vi "pulse from memory 16spc_v3.vi"(7 "stop this pulse":bool, 8 "run":bool=TRUE, 9 "referenses":T3={"clock x2"="IO Socket\\Data Clock 2x", "Memory In"="pulse on memory"}, 10 "start this pulse":bool, 11 "PDW":T1={"PW"=0, "frequency shift"=0.0, "amp"=0.9999923706054688, "mode type"=enum."CW", "mode depth"=0, "mode filter"=0, "phase shift"=0.0, "pulse shape filter"=0} {"frequency shift" format="%#_12f"}) -> (1 "free DDS":bool, 2 "output valid":bool=TRUE, 3 "IQ_out":T4[](array[typedef]))   [LabVIEW 2021]
uses:
  <instrlib>/_niInstr/DSP/v1/Shared/Public/IQ Data.ctl
  pulse_tx_vis/pdw.ctl
  pulse_tx_vis/CTL/mode_type.ctl
  <instrlib>/_niInstr/DSP/v1/FPGA/Public/Sub VIs/Data Conversion/U32 to IQ - 1 spc - S18.1.vi
  <instrlib>/FlexRIO/API/UsrFpgaDsp/v1/FPGA/HbInt/UsrFpgaDspHbIntIQ_8Cps_1xOC_BWper2_96dB.vi
  <instrlib>/FlexRIO/API/UsrFpgaDsp/v1/FPGA/HbInt/UsrFpgaDspHbIntIQ_4Cps_1xOC_BWper2_89dB.vi
  <instrlib>/FlexRIO/API/UsrFpgaDsp/v1/FPGA/HbInt/UsrFpgaDspHbIntIQ_2Cps_1xOC_BWper2_89dB.vi
  <vilib>/rvi/DataTransferAndStorage/Container/Common/niFpgaContainerExecOnDevCompGetState.vi
  <vilib>/rvi/Emulation/niFpgaEmulationIsFPGAContextNoSignature.vi
  <vilib>/rvi/DataTransferAndStorage/Container/Common/niFpgaContainerGetUniqueNameForEmu.vi
  <vilib>/rvi/Emulation/niFpgaProcessEmulError.vi
  <vilib>/rvi/Emulation/niFpgaSctlEmulationGetInTimedLoop.vi
  <vilib>/rvi/errors/nirviReportUnexpectedCaseInternalError (U32).vi
  <vilib>/rvi/Memory/Memory_Emulation/niFpgaMemoryEmulationCacheClearOnFirstRun.vi
  <vilib>/rvi/Memory/Memory_Emulation/nirvimemoryEmulationManagerCache_MakeExclusive.vi
  <vilib>/rvi/Memory/Memory_Emulation/niFpgaMemoryEmulationValidateCache.vi
  <vilib>/rvi/Memory/Memory_Emulation/nirvimemoryEmulationManagerCache_InsertValue.vi
  <vilib>/Utility/error.llb/Clear Errors.vi
  <vilib>/rvi/Memory/Memory_Emulation/nirvimemoryEmulationManagerCache_ReleaseExclusive.vi
  <vilib>/rvi/Memory/Memory_Emulation/nirvimemoryEmulationManagerCache_GetValue.vi
  <vilib>/rvi/Memory/Memory_Emulation/nirvimemoryEmulationManagerCache_SetValue.vi
  <vilib>/rvi/Emulation/niFpgaSctlEmulationResourceMgr.vi
  <instrlib>/FlexRIO/API/UsrFpgaDsp/v1/FPGA/HbInt/UsrFpgaDspHbIntIQ_1Spc_2xOC_BWper2_89dB.vi
  <instrlib>/FlexRIO/API/UsrFpgaDsp/v1/FPGA/HbInt/UsrFpgaDspHbIntIQ_2Spc_2xOC_BWper2_89dB.vi
  <instrlib>/FlexRIO/API/UsrFpgaDsp/v1/FPGA/HbInt/UsrFpgaDspHbIntIQ_4Spc_2xOC_BWper2_89dB.vi
  <instrlib>/FlexRIO/API/UsrFpgaDsp/v1/FPGA/HbInt/UsrFpgaDspHbIntIQ_8Spc_2xOC_BWper2_89dB.vi
  <instrlib>/_niInstr/DSP/v1/FPGA/Public/Sub VIs/Frequency Shift/Frequency Shift - 16 spc.vi
  <instrlib>/_niInstr/Basic Elements/v1/FPGA/Private/Count Up U32.vi
  <instrlib>/_niInstr/Basic Elements/v1/FPGA/Private/Count Up U16.vi
  <vilib>/rvi/DataTransferAndStorage/Container/XNode/niFpgaContainer.xnode
  <vilib>/rvi/Memory/Memory_Emulation/niFpgaMemoryEmulationRefIn.vi
  <instrlib>/_niInstr/DSP/v1/Shared/niInstr DSP v1 Shared.lvlib
  <instrlib>/_niInstr/DSP/v1/FPGA/niInstr DSP v1 FPGA.lvlib
  <instrlib>/_niInstr/Basic Elements/v1/FPGA/niInstr Basic Elements v1 FPGA.lvlib
  <instrlib>/FlexRIO/API/UsrFpgaDsp/v1/FPGA/HbInt/UsrFpgaDsp HbInt v1 FPGA.lvlib
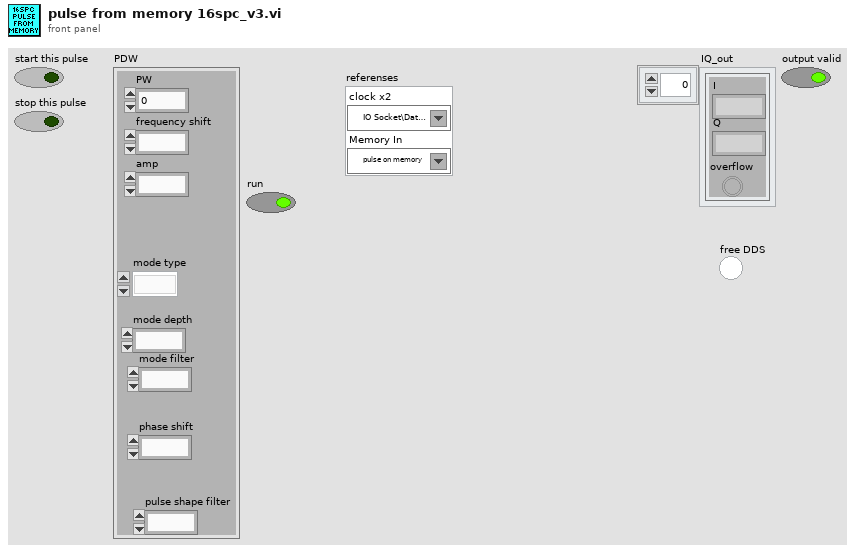
[diagram p1: front panel]
types:
  T1 = typedef "pdw.ctl" = cluster{"PW":u32, "frequency shift":fxp<+/-,48,0>, "amp":fxp<+/-,18,1>, "mode type":T2, "mode depth":u32, "mode filter":u8, "phase shift":fxp<+/-,16,1>, "pulse shape filter":u8}
  T2 = typedef "mode_type.ctl" = enum8{"CW", "from memory 1", "NC - cw", "LFM", "BPSK", "QPSK"}
  T3 = cluster{"clock x2":refnum<k21>, "Memory In":refnum<k21>}
  T4 = typedef "niInstr DSP v1 Shared.lvlib/IQ Data.ctl" = cluster{"I":fxp<+/-,18,1>, "Q":fxp<+/-,18,1>, "overflow":bool}
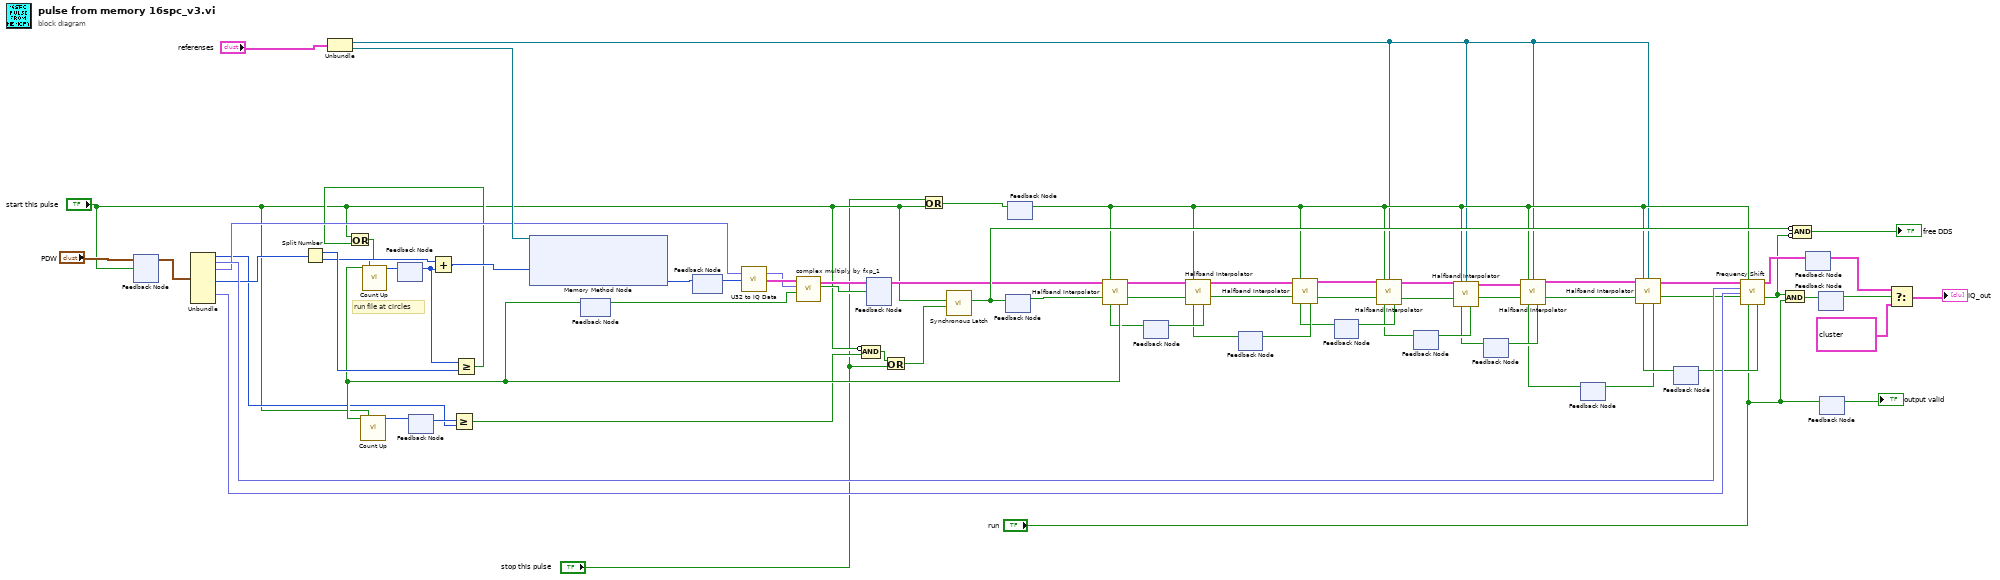
[diagram p0: block diagram]
diagram:
  # "run file at circles"
  n1 = feedback #1() -> (w65:T1)  [unwired: 1 in]
  n2 = feedback-in #1("PDW", "start this pulse") -> ()
  n3 = Unbundle(w65) -> ("PW"=w31:u32, "frequency shift"=w71:fxp<+/-,48,0>, "amp"=w59:fxp<+/-,18,1>, "mode depth"=w37:u32, "phase shift"=w70:fxp<+/-,16,1>)  [unwired: 3 out]
  n4 = Split Number(x=w37) -> (hi(x)=w64:u16, lo(x)=w58:u16)
  n5 = Unbundle("referenses") -> ("clock x2"=w13:refnum<k21>, "Memory In"=w67:refnum<k21>)
  n6 = feedback #2() -> (w56:u16)  [unwired: 1 in]
  n7 = feedback #3() -> (w32:u32)  [unwired: 1 in]
  n8 = Add(x=w58, y=w56) -> (x+y=w55:u16)
  n9 = Greater Or Equal?(x=w32, y=w31) -> (x >= y?=w30:bool)
  n10 = Greater Or Equal?(x=w56, y=w64) -> (x >= y?=w34:bool)
  n11 = Or(x="start this pulse", y=w34) -> (x .or. y?=w35:bool)
  n12 = xnode ("Memory Method Node")("Address"=w55, "Memory In"=w67) -> ("Data"=w74:u32)  [unwired: 1 out]
  n13 = feedback #4() -> (w60:bool)  [unwired: 1 in]
  n14 = feedback #5() -> (w73:u32)  [unwired: 1 in]
  n15 = feedback-in #5(w74) -> ()
  n16 = call-poly <instrlib>:"U32 to IQ Data.vi"("U32 data"=w73) -> ("IQ data"=w62:T4)  [unwired: 14 in]
  n17 = call "complex multiply by fxp_1.vi"("input valid"=w60, "amp"=w59, "IQ data"=w62) -> ("data valid"=w63:bool, "output cluster"=w61:T4)  [unwired: 7 in]
  n18 = Compound Arithmetic op=AND(invert "start this pulse", w30) -> (w3:bool)
  n19 = feedback #6() -> (w39:T4)  [unwired: 1 in]
  n20 = feedback-in #6(w61, w63) -> ()
  n21 = Or(x=w3, y="stop this pulse") -> (x .or. y?=w1:bool)
  n22 = Or(x="stop this pulse", y="start this pulse") -> (x .or. y?=w4:bool)
  n23 = call <instrlib>:"Synchronous Latch.vi"("clear"=w1, "set"="start this pulse") -> ("out"=w50:bool)  [unwired: 9 in]
  n24 = feedback #7() -> (w38:bool)  [unwired: 1 in]
  n25 = feedback-in #7(w50) -> ()
  n26 = feedback-in #8(w4) -> ()
  n27 = feedback #8() -> (w14:bool)  [unwired: 1 in]
  n28 = feedback #9() -> (w28:bool)  [unwired: 1 in]
  n29 = call-poly "Halfband Interpolator.vi"("data in"=w39, "reset"=w14, "input valid"=w38, "ready for output (T)"=w28) -> ("data out"=w49:T4, "output valid"=w40:bool, "ready for input"=w33:bool)  [unwired: 9 in]
  n30 = call-poly <instrlib>:"Count Up.vi"("increment"=w33, "reset"="start this pulse") -> ("count out"=w36:u32)  [unwired: 13 in]
  n31 = call-poly <instrlib>:"Count Up.vi"("increment"=w33, "reset"=w35) -> ("count out"=w57:u16)  [unwired: 13 in]
  n32 = feedback-in #2(w57) -> ()
  n33 = feedback-in #3(w36) -> ()
  n34 = feedback-in #4(w33) -> ()
  n35 = feedback #10() -> (w26:bool)  [unwired: 1 in]
  n36 = call-poly "Halfband Interpolator.vi"("data in"=w49, "reset"=w14, "input valid"=w40, "ready for output (T)"=w26) -> ("data out"=w48:T4, "output valid"=w41:bool, "ready for input"=w29:bool)  [unwired: 9 in]
  n37 = feedback-in #9(w29) -> ()
  n38 = feedback #11() -> (w24:bool)  [unwired: 1 in]
  n39 = call-poly "Halfband Interpolator.vi"("data in"=w48, "reset"=w14, "input valid"=w41, "ready for output (T)"=w24) -> ("data out"=w47:T4, "output valid"=w42:bool, "ready for input"=w27:bool)  [unwired: 9 in]
  n40 = feedback-in #10(w27) -> ()
  n41 = feedback #12() -> (w22:bool)  [unwired: 1 in]
  n42 = call-poly "Halfband Interpolator.vi"("data in"=w47, "reset"=w14, "clk2x"=w13, "input valid"=w42, "ready for output (T)"=w22) -> ("data out"=w46:T4[], "output valid"=w43:bool, "ready for input"=w25:bool)  [unwired: 8 in]
  n43 = feedback-in #11(w25) -> ()
  n44 = feedback #13() -> (w20:bool)  [unwired: 1 in]
  n45 = call-poly "Halfband Interpolator.vi"("data in"=w46, "reset"=w14, "clk2x"=w13, "input valid"=w43, "ready for output (T)"=w20) -> ("data out"=w45:T4[], "output valid"=w44:bool, "ready for input"=w23:bool)  [unwired: 8 in]
  n46 = feedback-in #12(w23) -> ()
  n47 = feedback #14() -> (w8:bool)  [unwired: 1 in]
  n48 = call-poly "Halfband Interpolator.vi"("data in"=w45, "reset"=w14, "clk2x"=w13, "input valid"=w44, "ready for output (T)"=w8) -> ("data out"=w12:T4[], "output valid"=w11:bool, "ready for input"=w21:bool)  [unwired: 8 in]
  n49 = feedback-in #13(w21) -> ()
  n50 = feedback #15() -> (w10:bool)  [unwired: 1 in]
  n51 = call-poly "Halfband Interpolator.vi"("data in"=w12, "reset"=w14, "clk2x"=w13, "input valid"=w11, "ready for output (T)"=w10) -> ("data out"=w7:T4[], "output valid"=w6:bool, "ready for input"=w9:bool)  [unwired: 8 in]
  n52 = feedback-in #14(w9) -> ()
  n53 = call-poly <instrlib>:"Frequency Shift.vi"("data in"=w7, "reset"=w14, "frequency shift"=w71, "phase"=w70, "input valid"=w6, "ready for output (T)"="run") -> ("data out"=w54:T4[], "output valid"=w17:bool, "ready for input"=w19:bool)  [unwired: 6 in, 1 out]
  n54 = feedback-in #15(w19) -> ()
  n55 = And(x=w17, y="run") -> (x .and. y?=w16:bool)
  n56 = Compound Arithmetic op=AND(invert w50, invert w17) -> (→"free DDS":bool)
  n57 = feedback #16() -> (w53:T4[])  [unwired: 1 in]
  n58 = feedback-in #16(w54) -> ()
  n59 = feedback #17() -> (w52:bool)  [unwired: 1 in]
  n60 = feedback-in #17(w16) -> ()
  n61 = feedback #18() -> (→"output valid":bool)  [unwired: 1 in]
  n62 = feedback-in #18("run") -> ()
  n63 = Select(t=w53, s=w52, f=T4[] [{"I"=0.0, "Q"=0.0, "overflow"=FALSE}, {"I"=0.0, "Q"=0.0, "overflow"=FALSE}, {"I"=0.0, "Q"=0.0, "overflow"=FALSE}, {"I"=0.0, "Q"=0.0, "overflow"=FALSE}, {"I"=0.0, "Q"=0.0, "overflow"=FALSE}, {"I"=0.0, "Q"=0.0, "overflow"=FALSE}, {"I"=0.0, "Q"=0.0, "overflow"=FALSE}, {"I"=0.0, "Q"=0.0, "overflow"=FALSE}, {"I"=0.0, "Q"=0.0, "overflow"=FALSE}, {"I"=0.0, "Q"=0.0, "overflow"=FALSE}, {"I"=0.0, "Q"=0.0, "overflow"=FALSE}, {"I"=0.0, "Q"=0.0, "overflow"=FALSE}, {"I"=0.0, "Q"=0.0, "overflow"=FALSE}, {"I"=0.0, "Q"=0.0, "overflow"=FALSE}, {"I"=0.0, "Q"=0.0, "overflow"=FALSE}, {"I"=0.0, "Q"=0.0, "overflow"=FALSE}] ("data out")) -> (s? t:f=→"IQ_out":T4[])
